vi "init.vi"(8 "error in":errorcluster, 11 "Which Data Technique":T2) -> (0 "error out":errorcluster, 3 "cycle results cluster input":T1)   [LabVIEW 2016]
uses:
  controls/cycle results control.ctl
  controls/sequence calculation technique.ctl
  controls/cycle sort control.ctl
  controls/unique results control.ctl
panel:
  out "cycle results cluster result":T1 {"cycle results dbl" format="%#_6e"}
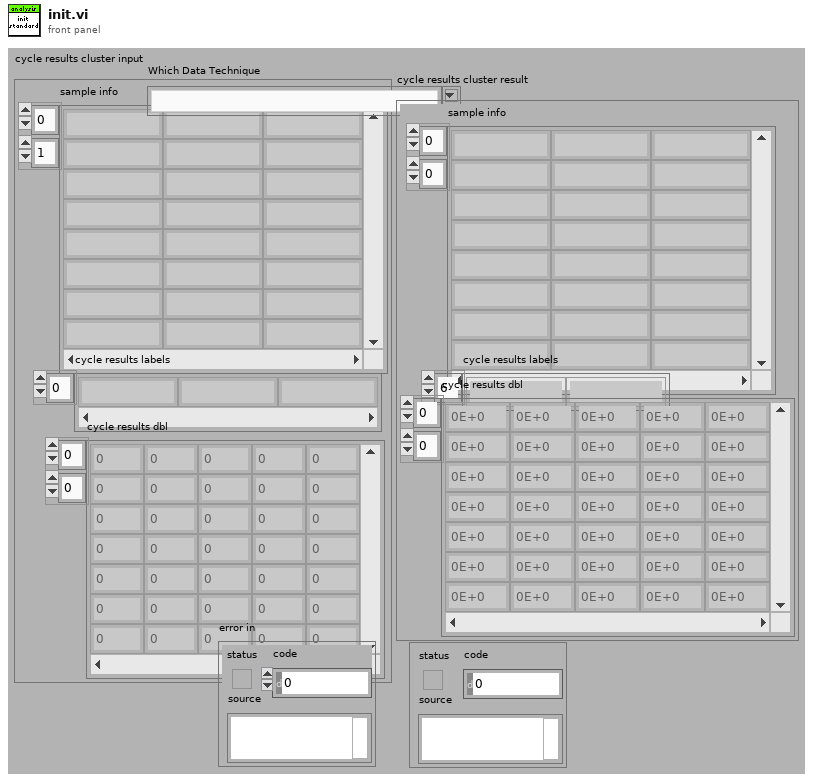
[diagram p1: front panel]
types:
  T1 = typedef "cycle results control.ctl" = cluster{"sample info":string[][], "cycle results labels":string[], "cycle results dbl":dbl[][]}
  T2 = typedef "sequence calculation technique.ctl" = string
  T3 = typedef "unique results control.ctl" = string
  T4 = typedef "cycle sort control.ctl" = string
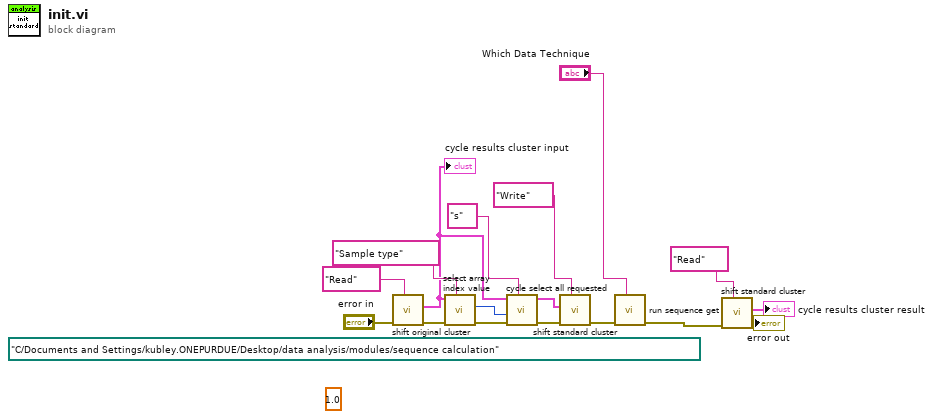
[diagram p0: block diagram]
diagram:
  (unwired) path "C:/Documents and Settings/kubley.ONEPURDUE/Desktop/data analysis/modules/sequence calculation" ("path")
  (unwired) 1.0 ("y")
  n1 = call "shift original cluster.vi"("read write shift"="Read", "error in"="error in") -> ("error out"=w3:errorcluster, "cycle results cluster out"=w7:T1)  [unwired: 8 in]
  "cycle results cluster input" <- w7
  n2 = call "select array index value.vi"("Sort by which item"=T4 "Sample type", "error in"=w3, "cycle results cluster"=w7) -> ("error out"=w8:errorcluster, "value that will be sorted"=w14:i32)  [unwired: 6 in, 1 out]
  n3 = call "cycle select all requested.vi"("which value to be selected"=T3 "s", "error in"=w8, "value that will be sorted In"=w14, "cycle results cluster IN"=w7) -> ("error out"=w16:errorcluster, "cycle results cluster out"=w1:T1)  [unwired: 6 in]
  n4 = call "shift standard cluster.vi"("read write shift"="Write", "error in"=w16, "cycle results cluster In"=w1) -> ("error out"=w11:errorcluster)  [unwired: 7 in, 1 out]
  n5 = call "run sequence get.vi"("Which Data Technique"="Which Data Technique", "error in"=w11) -> ("error out"=w6:errorcluster)  [unwired: 8 in, 1 out]
  n6 = call "shift standard cluster.vi"("read write shift"="Read", "error in"=w6) -> ("error out"=→"error out":errorcluster, "cycle results cluster out"=→"cycle results cluster result":T1)  [unwired: 8 in]
